vi "PDCMeansOfSplitImages.vi"(11 "ImageData":u16[](array[numeric])) -> (3 "MeansOfSplitImages":dbl[](array[numeric]))   [LabVIEW 2015]
uses:
  <vilib>/Analysis/baseanly.llb/Mean (DBL).vi
  <vilib>/Analysis/NI_AALBase.lvlib
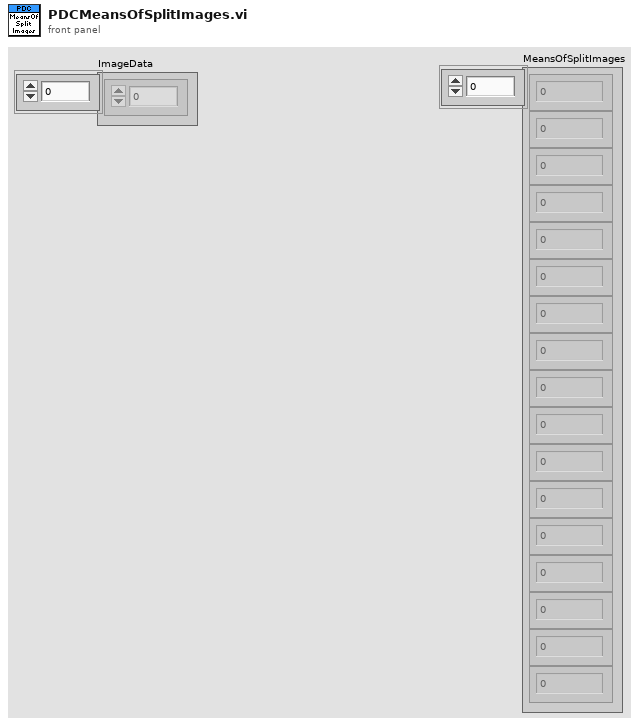
[diagram p1: front panel]
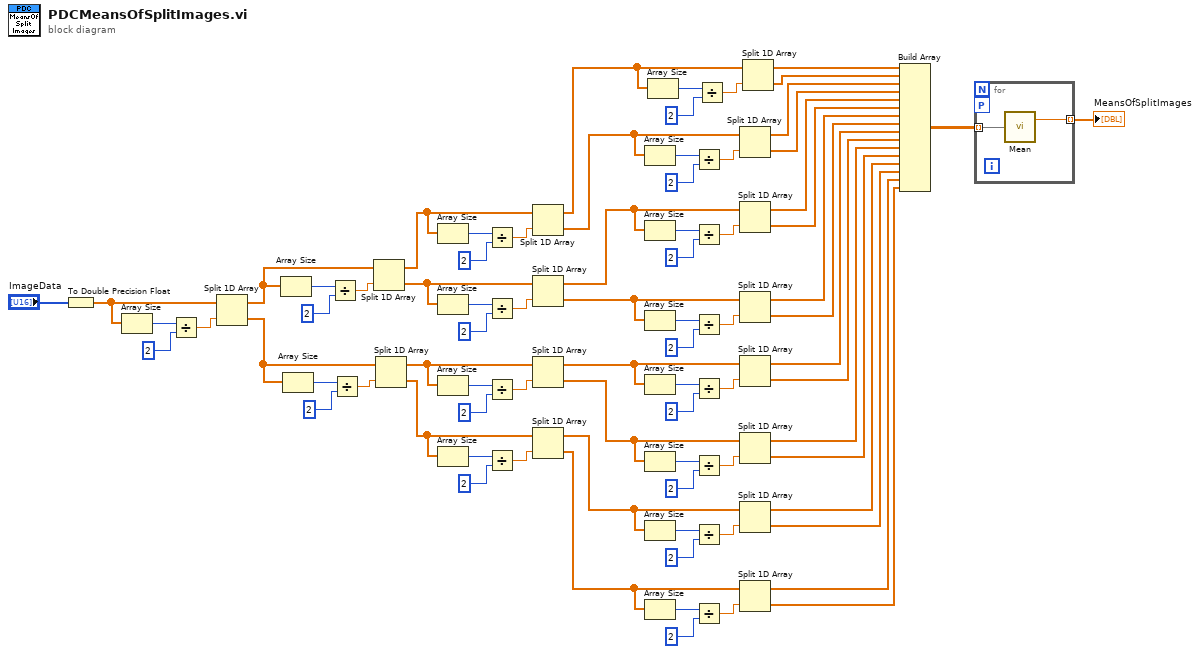
[diagram p0: block diagram]
diagram:
  n1 = To Double Precision Float(number="ImageData") -> (double precision float=w51:dbl[])
  n2 = Array Size(array=w51) -> (size(s)=w54:i32)
  n3 = Divide(x=w54, y=2) -> (x/y=w55:dbl)
  n4 = Split 1D Array(array=w51, index=w55) -> (first subarray=w63:dbl[], second subarray=w62:dbl[])
  n5 = Array Size(array=w63) -> (size(s)=w56:i32)
  n6 = Array Size(array=w62) -> (size(s)=w61:i32)
  n7 = Divide(x=w56, y=2) -> (x/y=w58:dbl)
  n8 = Divide(x=w61, y=2) -> (x/y=w59:dbl)
  n9 = Split 1D Array(array=w63, index=w58) -> (first subarray=w67:dbl[], second subarray=w71:dbl[])
  n10 = Split 1D Array(array=w62, index=w59) -> (first subarray=w78:dbl[], second subarray=w79:dbl[])
  n11 = Array Size(array=w67) -> (size(s)=w65:i32)
  n12 = Array Size(array=w71) -> (size(s)=w69:i32)
  n13 = Array Size(array=w78) -> (size(s)=w76:i32)
  n14 = Array Size(array=w79) -> (size(s)=w73:i32)
  n15 = Divide(x=w65, y=2) -> (x/y=w64:dbl)
  n16 = Divide(x=w69, y=2) -> (x/y=w70:dbl)
  n17 = Divide(x=w76, y=2) -> (x/y=w77:dbl)
  n18 = Divide(x=w73, y=2) -> (x/y=w72:dbl)
  n19 = Split 1D Array(array=w67, index=w64) -> (first subarray=w26:dbl[], second subarray=w25:dbl[])
  n20 = Split 1D Array(array=w71, index=w70) -> (first subarray=w24:dbl[], second subarray=w23:dbl[])
  n21 = Split 1D Array(array=w78, index=w77) -> (first subarray=w22:dbl[], second subarray=w21:dbl[])
  n22 = Split 1D Array(array=w79, index=w72) -> (first subarray=w19:dbl[], second subarray=w20:dbl[])
  n23 = Array Size(array=w25) -> (size(s)=w46:i32)
  n24 = Array Size(array=w24) -> (size(s)=w43:i32)
  n25 = Array Size(array=w23) -> (size(s)=w40:i32)
  n26 = Array Size(array=w22) -> (size(s)=w37:i32)
  n27 = Array Size(array=w21) -> (size(s)=w34:i32)
  n28 = Array Size(array=w19) -> (size(s)=w31:i32)
  n29 = Array Size(array=w20) -> (size(s)=w28:i32)
  n30 = Array Size(array=w26) -> (size(s)=w49:i32)
  n31 = Divide(x=w46, y=2) -> (x/y=w47:dbl)
  n32 = Divide(x=w43, y=2) -> (x/y=w42:dbl)
  n33 = Divide(x=w40, y=2) -> (x/y=w41:dbl)
  n34 = Divide(x=w37, y=2) -> (x/y=w36:dbl)
  n35 = Divide(x=w34, y=2) -> (x/y=w35:dbl)
  n36 = Divide(x=w31, y=2) -> (x/y=w30:dbl)
  n37 = Divide(x=w28, y=2) -> (x/y=w29:dbl)
  n38 = Divide(x=w49, y=2) -> (x/y=w48:dbl)
  n39 = Split 1D Array(array=w25, index=w47) -> (first subarray=w16:dbl[], second subarray=w15:dbl[])
  n40 = Split 1D Array(array=w24, index=w42) -> (first subarray=w14:dbl[], second subarray=w13:dbl[])
  n41 = Split 1D Array(array=w23, index=w41) -> (first subarray=w12:dbl[], second subarray=w11:dbl[])
  n42 = Split 1D Array(array=w22, index=w36) -> (first subarray=w10:dbl[], second subarray=w9:dbl[])
  n43 = Split 1D Array(array=w21, index=w35) -> (first subarray=w8:dbl[], second subarray=w7:dbl[])
  n44 = Split 1D Array(array=w19, index=w30) -> (first subarray=w6:dbl[], second subarray=w5:dbl[])
  n45 = Split 1D Array(array=w20, index=w29) -> (first subarray=w4:dbl[], second subarray=w3:dbl[])
  n46 = Split 1D Array(array=w26, index=w48) -> (first subarray=w18:dbl[], second subarray=w17:dbl[])
  n47 = Build Array(w18, w17, w16, w15, w14, w13, w12, w11, w10, w9, w8, w7, w6, w5, w4, w3) -> (w2:dbl[][])
  n48 = for {
    tunnel: w2 -> [w81] mode=indexing
    tunnel: [w80] -> w1 mode=indexing
    workers-P: _ -> [_]
    n49 = call-poly <vilib>:"Mean.vi"("X"=w81) -> ("mean"=w80:dbl)  [unwired: 1 out]
  }
  "MeansOfSplitImages" <- w1
